vi "NF WF1973_74 TRIG Sour.vi"(6 "Read(F)":bool, 7 "Set(Sweep)":bool, 8 "error in (no error)":errorcluster caption="Error IN", 9 "Source(Timer)":u32(ring) items=["Timer", "External", "CH1"], 10 "Ch(Ch1)":bool, 11 "VISAsession":refnum<visa-resource-name>) -> (0 "error out":errorcluster caption="Error OUT", 2 "Query Source":string, 3 "CopyVISAsession":refnum<visa-resource-name>)   [LabVIEW 2010]
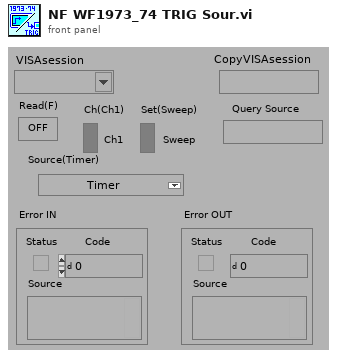
[diagram p1: front panel]
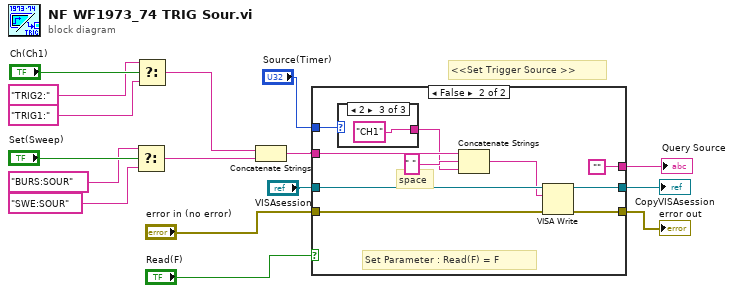
[diagram p0: block diagram]
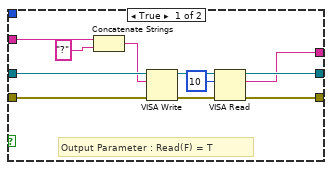
[diagram p2: hidden frame]
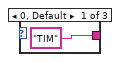
[diagram p3: hidden frame]
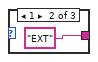
[diagram p4: hidden frame]
diagram:
  # "<<Set Trigger Source >>"
  n1 = Select(t="BURS:SOUR", s="Set(Sweep)", f="SWE:SOUR") -> (s? t:f=w1:string)
  n2 = Select(t="TRIG2:" ("文字列"), s="Ch(Ch1)", f="TRIG1:" ("文字列")) -> (s? t:f=w2:string)
  n3 = Concatenate Strings(w2, w1) -> (w3:string)
  n4 = case shown="FALSE" "Read(F)" {
    tunnel: "VISAsession" -> [w27 w37]
    tunnel: [w24 w35] -> w15
    tunnel: [w23 w36] -> w14
    tunnel: "error in (no error)" -> [w22 w29]
    tunnel: w3 -> [w20 w32]
    tunnel: "Source(Timer)" -> [_ w31]
    tunnel: [w17 ""] -> w10
    frame True {
      # "Output Parameter : Read(F) = T"
      n5 = Concatenate Strings(w20, "?" ("形式文字列")) -> (w18:string)
      n6 = VISA Write(VISA resource name=w27, write buffer=w18, error in (no error)=w22) -> (VISA resource name out=w25:refnum<visa-resource-name>, error out=w26:errorcluster)  [unwired: 1 out]
      n7 = VISA Read(VISA resource name=w25, byte count=u32 10 ("バイトカウント（0）"), error in (no error)=w26) -> (VISA resource name out=w24:refnum<visa-resource-name>, read buffer=w17:string, error out=w23:errorcluster)  [unwired: 1 out]
    }
    frame False {
      # "space"
      # "Set Parameter : Read(F) = F"
      n8 = case shown="2" w31 {
        tunnel: ["TIM" "EXT" "CH1"] -> w30
        frame 0, Default {
        }
        frame 1 {
        }
        frame 2 {
        }
      }
      n9 = Concatenate Strings(w32, " ", w30) -> (w34:string)
      n10 = VISA Write(VISA resource name=w37, write buffer=w34, error in (no error)=w29) -> (VISA resource name out=w35:refnum<visa-resource-name>, error out=w36:errorcluster)  [unwired: 1 out]
    }
  }
  "error out" <- w14
  "CopyVISAsession" <- w15
  "Query Source" <- w10
